vi "CheckFoderExists.vi"(8 "error in (no error)":errorcluster, 10 "shotnumber":i32, 11 "Input Stripped Path":path) -> (0 "error out":errorcluster)   [LabVIEW 2020, in "BaseDriver.lvclass"]
uses:
  BaseDriver.lvclass
panel:
  out "Execution Time":u32
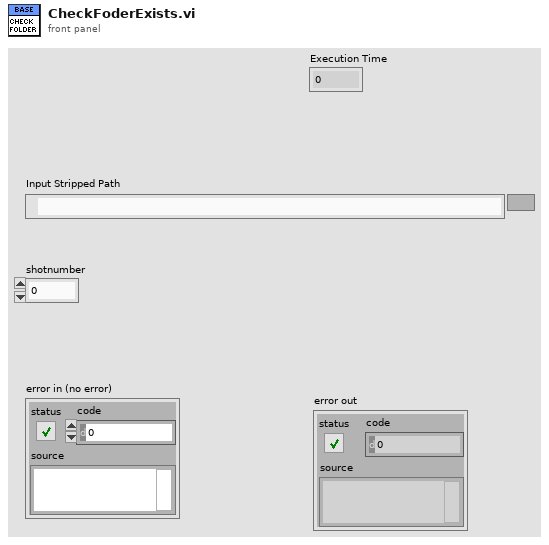
[diagram p1: front panel]
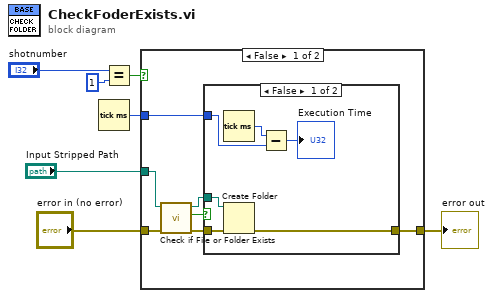
[diagram p0: block diagram]
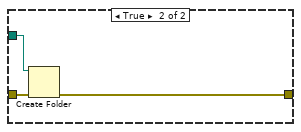
[diagram p3: hidden frame]
diagram:
  n1 = Tick Count (ms)() -> (millisecond timer value=w1:u32)
  n2 = Equal?(x="shotnumber", y=1) -> (x = y?=w5:bool)
  n3 = case shown="False" w5 {
    tunnel: "Input Stripped Path" -> [w10 w24]
    tunnel: "error in (no error)" -> [w14 w23]
    tunnel: [w11 w22] -> w2
    tunnel: w1 -> [w8 _]
    frame False {
      n4 = call "Check if File or Folder Exists.vi"("error in (no error)"=w14, "path"=w10) -> ("error out"=w12:errorcluster, "file or folder exists?"=w13:bool, "dup path"=w9:path)  [unwired: 7 out]
      n5 = case shown="False" w13 {
        tunnel: w12 -> [w20 w21]
        tunnel: [w19 w21] -> w11
        tunnel: w9 -> [w18 _]
        tunnel: w8 -> [w16 _]
        frame False {
          n6 = Tick Count (ms)() -> (millisecond timer value=w17:u32)
          n7 = Create Folder(path (use dialog)=w18, error in=w20) -> (error out=w19:errorcluster)  [unwired: 3 out]
          n8 = Subtract(x=w17, y=w16) -> (x-y=→"Execution Time":u32)
        }
        frame True {
        }
      }
    }
    frame True {
      n9 = Create Folder(path (use dialog)=w24, error in=w23) -> (error out=w22:errorcluster)  [unwired: 3 out]
    }
  }
  "error out" <- w2
